vi "hmi_roller.vi"(11 "UserData":T1) -> ()   [LabVIEW 2011]
uses:
  user_data.ctl
  user_buttons_dualaction.ctl
  user_buttons_360.ctl
  roller/roller_user_state.ctl
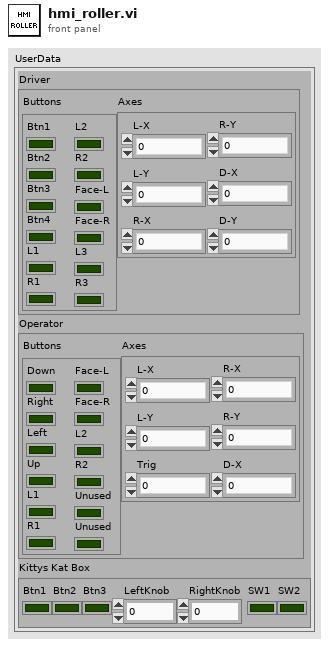
[diagram p1: front panel]
types:
  T1 = typedef "user_data.ctl" = cluster{"Driver":cluster{"Buttons":T2, "Axes":cluster{"L-X":dbl, "L-Y":dbl, "R-X":dbl, "R-Y":dbl, "D-X":dbl, "D-Y":dbl}}, "Operator":cluster{"Buttons":T3, "Axes":cluster{"L-X":dbl, "L-Y":dbl, "Trig":dbl, "R-X":dbl, "R-Y":dbl, "D-X":dbl}}, "Kittys Kat Box":cluster{"Btn1":bool, "Btn2":bool, "Btn3":bool, "LeftKnob":dbl, "RightKnob":dbl, "SW1":bool, "SW2":bool}}
  T2 = typedef "user_buttons_dualaction.ctl" = cluster{"Btn1":bool, "Btn2":bool, "Btn3":bool, "Btn4":bool, "L1":bool, "R1":bool, "L2":bool, "R2":bool, "Face-L":bool, "Face-R":bool, "L3":bool, "R3":bool}
  T3 = typedef "user_buttons_360.ctl" = cluster{"Down":bool, "Right":bool, "Left":bool, "Up":bool, "L1":bool, "R1":bool, "Face-L":bool, "Face-R":bool, "L2":bool, "R2":bool, "Unused":bool, "Unused":bool}
  T4 = typedef "roller_user_state.ctl" = enum16{"off", "collect", "blow", "force suck"}
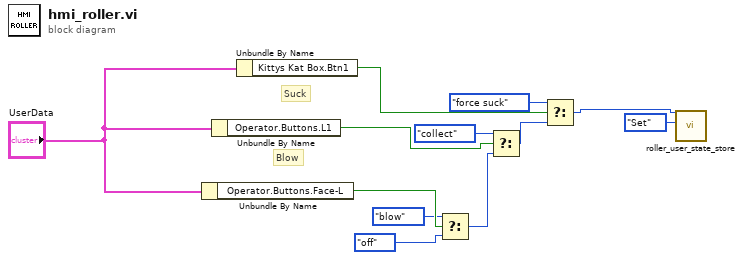
[diagram p0: block diagram]
diagram:
  # "Blow"
  # "Suck"
  n1 = Unbundle By Name("UserData") -> ("Operator.Buttons.Face-L"=w9:bool)
  n2 = Unbundle By Name("UserData") -> ("Operator.Buttons.L1"=w12:bool)
  n3 = Unbundle By Name("UserData") -> ("Kittys Kat Box.Btn1"=w2:bool)
  n4 = Select(t=roller_user_state."blow", s=w9, f=roller_user_state."off" ("roller user state")) -> (s? t:f=w10:T4)
  n5 = Select(t=roller_user_state."collect", s=w12, f=w10) -> (s? t:f=w5:T4)
  n6 = Select(t=roller_user_state."force suck", s=w2, f=w5) -> (s? t:f=w4:T4)
  n7 = call "roller_user_state_store.vi"("data_store_mode"=enum16{"Set", "Get"}."Set", "roller user state"=w4) -> ()  [unwired: 9 in, 1 out]
